vi "Get Username.vi"(8 "error in (no error)":errorcluster, 11 "File Transfer Behavior in":refnum<class "File Transfer Behavior.lvclass">) -> (0 "error out":errorcluster, 2 "Username":string, 3 "File Transfer Behavior out":refnum<class "File Transfer Behavior.lvclass">)   [LabVIEW 2015, in "RT Management.lvlib" / "File Transfer Behavior.lvclass"]
uses:
  File Transfer Behavior.lvclass
  File Transfer Behavior.lvclass/File Transfer Behavior.ctl
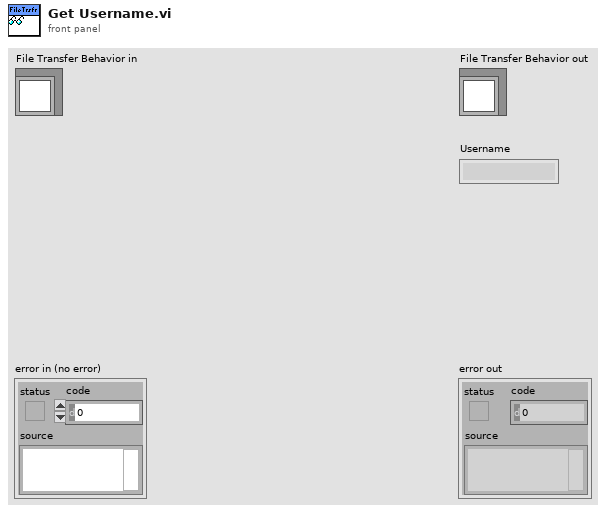
[diagram p1: front panel]
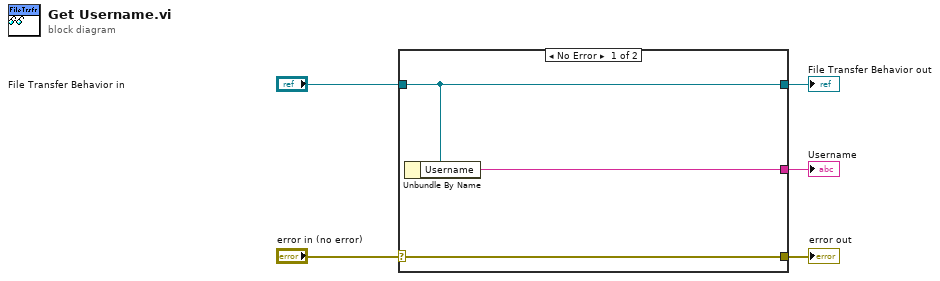
[diagram p0: block diagram]
diagram:
  n1 = case shown="No Error" "error in (no error)" {
    selector: "error in (no error)" -> [w8 w9]
    tunnel: [w8 w9] -> w4
    tunnel: [w7 w10] -> w2
    tunnel: "File Transfer Behavior in" -> [w7 w10]
    tunnel: [w6 _] -> w1
    frame No Error {
      n2 = Unbundle By Name(w7) -> ("Username"=w6:string)
    }
    frame Error {
    }
  }
  "error out" <- w4
  "File Transfer Behavior out" <- w2
  "Username" <- w1
